vi "RSZVB Set Remote Language.vi"(8 "error in (no error)":errorcluster {"code" format="%.0x"}, 10 "Language (0: SCPI)":i32(ring) items=["SCPI", "PNA", "HP8510", "HP8720", "HP8753"], 11 "VISA session":refnum<visa-resource-name>) -> (0 "error out":errorcluster {"code" format="%.0x"}, 3 "dup VISA session":refnum<visa-resource-name>)   [LabVIEW 2011]
doc: "This VI specifies the Remote Language for the analyzer.\n\nRemote-control command(s):\nSYSTem:LANGuage 'SCPI' | 'PNA' | 'HP8510' | 'HP8720' | 'HP8753'"
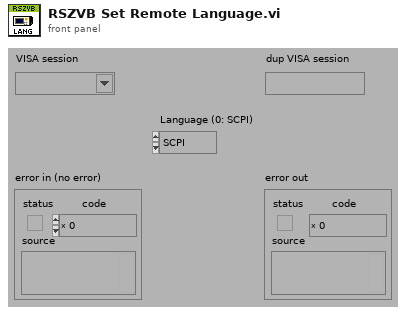
[diagram p1: front panel]
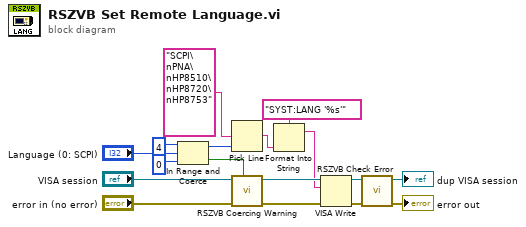
[diagram p0: block diagram]
diagram:
  n1 = In Range and Coerce(upper limit=4, x="Language (0: SCPI)", lower limit=0) -> (coerced(x)=w7:i32, In Range?=w11:bool)
  n2 = Pick Line(multi-line string="SCPI\nPNA\nHP8510\nHP8720\nHP8753", line index=w7) -> (output string=w5:string)  [unwired: 1 in]
  n3 = call "RSZVB Coercing Warning.vi"("In Range?"=w11, "error in (no error)"="error in (no error)", "VISA session"="VISA session") -> ("error out"=w15:errorcluster, "dup VISA session"=w16:refnum<visa-resource-name>)  [unwired: 7 in]
  n4 = Format Into String(format string="SYST:LANG '%s'", w5) -> (resulting string=w12:string)  [unwired: 2 in, 1 out]
  n5 = VISA Write(VISA resource name=w16, write buffer=w12, error in (no error)=w15) -> (VISA resource name out=w13:refnum<visa-resource-name>, error out=w14:errorcluster)  [unwired: 1 out]
  n6 = call "RSZVB Check Error.vi"("error in (no error)"=w14, "VISA session"=w13) -> ("error out"=→"error out":errorcluster, "dup VISA session"=→"dup VISA session":refnum<visa-resource-name>)  [unwired: 8 in]
